vi "solar_visa Query (Simulate).vi"(7 "Action (Get)":enum8{"Get", "Set", "Clear"}(ring), 8 "error in (no error)":errorcluster, 10 "Next SCPI Response":string, 11 "VISA Resource in":refnum<visa-resource-name>) -> (0 "error out":errorcluster, 2 "SCPI Response (Latching)":string, 3 "VISA Resource out":refnum<visa-resource-name>)   [LabVIEW 2018]
doc: "This VISA simulator stores the next expect response back from the VISA resource. Set the <b>Next Response</b> to query the next time the Get action is called."
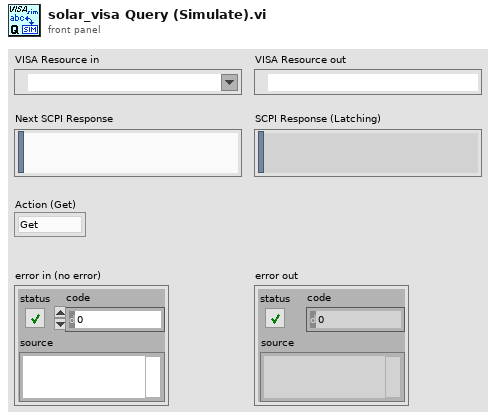
[diagram p1: front panel]
types:
  T1 = cluster{"Responses":string[], "LastResp":string}[]
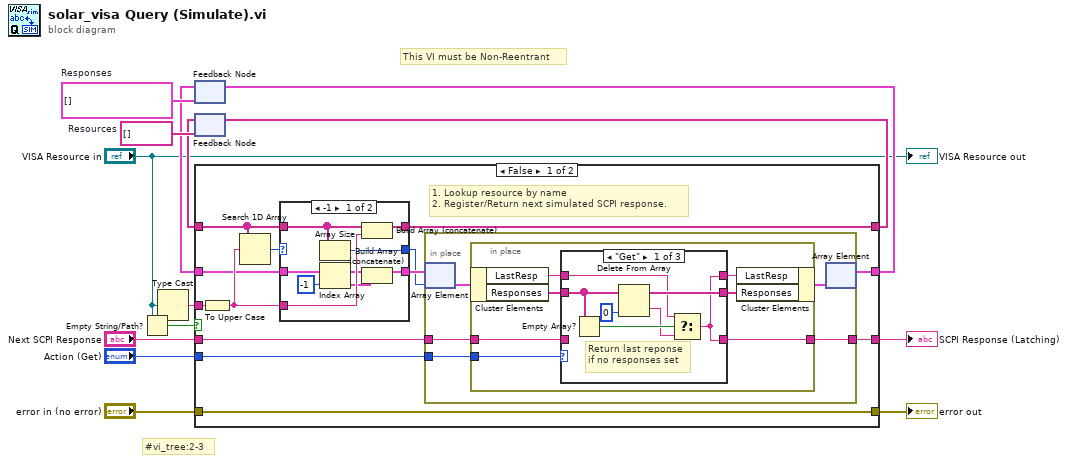
[diagram p0: block diagram]
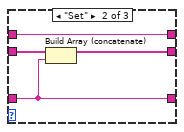
[diagram p2: hidden frame]
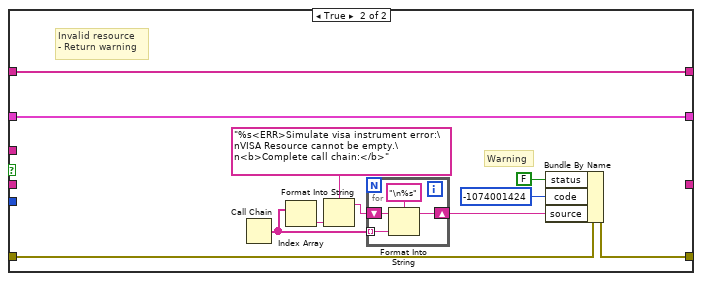
[diagram p5: hidden frame]
diagram:
  w11 = T1 []  # Responses
  w14 = string[] []  # Resources
  # "#vi_tree:2-3"
  # "This VI must be Non-Reentrant"
  n1 = Empty String/Path?(string/path="VISA Resource in") -> (empty?=w4:bool)
  n2 = Type Cast(x="VISA Resource in") -> (*(type *) &x=w13:string)  [unwired: 1 in]
  n3 = feedback #1(w11) -> (w10:T1)
  n4 = feedback #2(w14) -> (w12:string[])
  n5 = case shown="False" w4 {
    tunnel: w13 -> [w27 _]
    tunnel: w12 -> [w24 w73]
    tunnel: w10 -> [w23 w72]
    tunnel: "Action (Get)" -> [w16 _]
    tunnel: [w21 w72] -> w8
    tunnel: [w17 w73] -> w7
    tunnel: "Next SCPI Response" -> [w20 _]
    tunnel: [w18 _] -> w1
    tunnel: [w15 w63] -> w2
    tunnel: "error in (no error)" -> [w15 w64]
    frame False {
      # "1. Lookup resource by name\n2. Register/Return next simulated SCPI response."
      n6 = To Upper Case(1:w27) -> (0:w25:string)
      n7 = Search 1D Array(1D array=w24, element=w25) -> (index of element=w26:i32)  [unwired: 1 in]
      n8 = case shown="-1" w26 {
        selector: w26 -> [_ w60]
        tunnel: w25 -> [w58 _]
        tunnel: w24 -> [w53 w61]
        tunnel: w23 -> [w56 w62]
        tunnel: [w57 w62] -> w22
        tunnel: [w59 w61] -> w17
        tunnel: [w52 w60] -> w19
        frame -1 {
          n9 = Array Size(array=w53) -> (size(s)=w52:i32)
          n10 = Index Array(array=w56, index=-1) -> (element=w55:cluster{"Responses":string[], "LastResp":string})
          n11 = Build Array (concatenate)(w53, w58) -> (w59:string[])
          n12 = Build Array (concatenate)(w56, w55) -> (w57:T1)
        }
        frame Default {
        }
      }
      n13 = in-place {
        in-place-border: w20 -> [w32]
        in-place-border: [w30] -> w18
        in-place-border: w16 -> [w29]
        n14 = in-place-array #3(w22, w19) -> (w31:cluster{"Responses":string[], "LastResp":string})
        n15 = in-place {
          in-place-border: w32 -> [w37]
          in-place-border: [w35] -> w30
          in-place-border: w29 -> [w36]
          n16 = in-place-cluster #4(w31) -> ("LastResp"=w33:string, "Responses"=w39:string[])
          n17 = case shown="\"Get\"" w36 {
            tunnel: w39 -> [w44 w50 _]
            tunnel: [w46 w49 _] -> w38
            tunnel: w37 -> [_ w48 w51]
            tunnel: [w40 w48 w51] -> w35
            tunnel: [w40 w47 w51] -> w34
            tunnel: w33 -> [w42 w47 _]
            frame "Get" {
              # "Return last reponse\nif no responses set"
              n18 = Empty Array?(array=w44) -> (empty?=w43:bool)
              n19 = Delete From Array(array=w44, index=0) -> (deleted portion=w41:string, array with subset deleted=w46:string[])  [unwired: 1 in]
              n20 = Select(t=w42, s=w43, f=w41) -> (s? t:f=w40:string)
            }
            frame "Set" {
              n21 = Build Array (concatenate)(w50, w48) -> (w49:string[])
            }
            frame "Clear" {
            }
          }
          n22 = in-place-cluster #4("LastResp"=w34, "Responses"=w38) -> (w28:cluster{"Responses":string[], "LastResp":string})
        }
        n23 = in-place-array #3(w28) -> (w21:T1)  [unwired: 1 out]
      }
    }
    frame True {
      # "Warning"
      # "Invalid resource\n- Return warning"
      n24 = Call Chain() -> (call chain=w66:string[])
      n25 = Index Array(array=w66) -> (element=w68:string)  [unwired: 1 in]
      n26 = Format Into String(format string="%s<ERR>Simulate visa instrument error:\nVISA Resource cannot be empty.\n<b>Complete call chain:</b>", w68) -> (resulting string=w67:string)  [unwired: 2 in, 1 out]
      n27 = for {
        tunnel: w66 -> [w77] mode=indexing
        shift-right: [w76] -> w65
        shift-left: w67 -> [w75]
        n28 = Format Into String(format string="\n%s", initial string=w75, w77) -> (resulting string=w76:string)  [unwired: 1 in, 1 out]
      }
      n29 = Bundle By Name(cluster=w64, "status"=FALSE, "code"=-1074001424 ("Code"), "source"=w65) -> (w63:errorcluster)
    }
  }
  "error out" <- w2
  "SCPI Response (Latching)" <- w1
  n30 = feedback-in #1(w8) -> ()
  n31 = feedback-in #2(w7) -> ()
  "VISA Resource out" <- "VISA Resource in"
